vi "init.vi"(8 "error in (no error)":errorcluster, 11 "CL57RS in":refnum<class "CL57RS.lvclass">) -> (0 "error out":errorcluster, 3 "CL57RS out":refnum<class "CL57RS.lvclass">)   [LabVIEW 2025, in "Motor.lvlib" / "CL57RS.lvclass"]
uses:
  CL57RS.lvclass
  CL57RS.lvclass/CL57RS.ctl
  <vilib>/NI/Modbus Library/API/Wrapper/Create Serial Master.vi
  <vilib>/NI/Modbus Library/API/Wrapper/API Main.lvlib
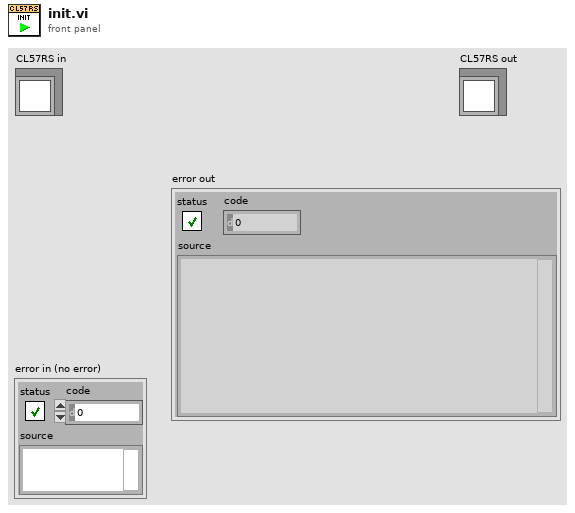
[diagram p1: front panel]
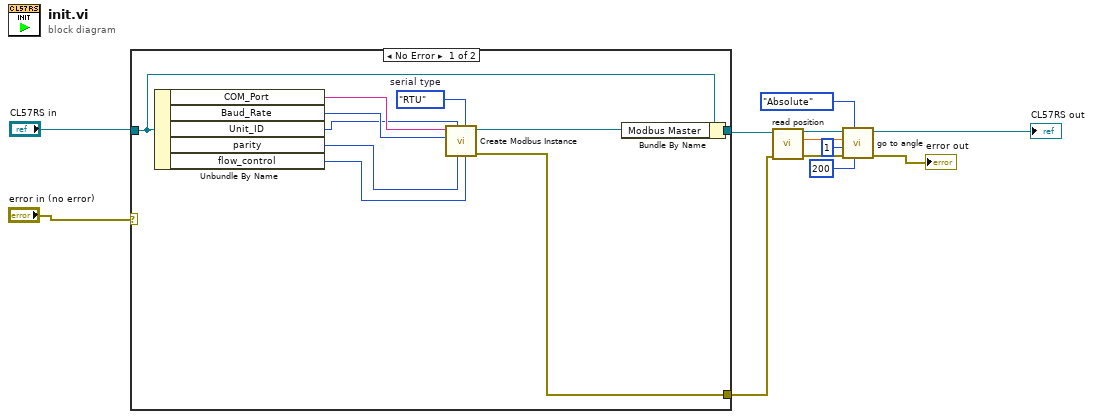
[diagram p0: block diagram]
diagram:
  n1 = case shown="No Error" "error in (no error)" {
    selector: "error in (no error)" -> [_ w24]
    tunnel: [w13 w24] -> w9
    tunnel: [w22 w23] -> w10
    tunnel: "CL57RS in" -> [w21 w23]
    frame No Error {
      w17 = enum16{"RTU", "ASCII"}."RTU"  # serial type
      n2 = Unbundle By Name(w21) -> ("COM_Port"=w20:string, "Baud_Rate"=w19:u32, "Unit_ID"=w18:u8, "parity"=w16:u16, "flow_control"=w15:u16)
      n3 = call-poly <vilib>:"Create Modbus Instance.vi"("flow control (none)"=w15, "serial type"=w17, "parity (even)"=w16, "unit ID"=w18, "baud rate"=w19, "VISA resource name"=w20) -> ("error out"=w13:errorcluster, "serial master instance"=w14:refnum<class "Modbus Master.lvclass">)  [unwired: 4 in]
      n4 = Bundle By Name(cluster=w21, "Modbus Master"=w14) -> (w22:refnum<class "CL57RS.lvclass">)
    }
    frame Error {
    }
  }
  n5 = call-dynamic "read position.vi"("error in (no error)"=w9, "CL57RS in"=w10) -> ("error out"=w8:errorcluster, "Angle"=w7:dbl, "CL57RS out"=w5:refnum<class "CL57RS.lvclass">)  [unwired: 7 in]
  n6 = call-dynamic "go to angle.vi"("Pause Time [ms]"=200, "Relative?"=enum16{"Relative", "Absolute"}."Absolute", "error in (no error)"=w8, "Velocity [rpm]"=1, "Angle"=w7, "CL57RS in"=w5) -> ("error out"=→"error out":errorcluster, "CL57RS out"=→"CL57RS out":refnum<class "CL57RS.lvclass">)  [unwired: 4 in]
